vi "status_machine_value.vi"(8 "Main_Status_in":T2, 9 "Main상태쓰기":bool, 10 "Vesa_Status_in":T1, 11 "vesa상태쓰기":bool) -> (0 "Main Exit?":bool, 1 "Main_Status":T2, 2 "DisConnect?":bool, 3 "Vesa_Status":T1)   [LabVIEW 2014]
uses:
  VESA_Status.ctl
  Main_status.ctl
  bus_button.xctl
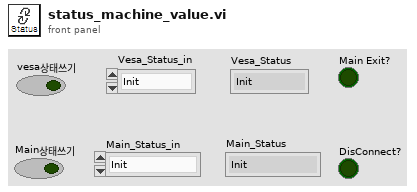
[diagram p1: front panel]
types:
  T1 = typedef "bus_button.xctl/VESA_Status.ctl" = enum16{"Init", "Wait", "Connect", "DisConnect", "Idel", "Exit"}
  T2 = typedef "Main_status.ctl" = enum16{"Init", "Wait", "connect", "Idle", "disc", "Exit"}
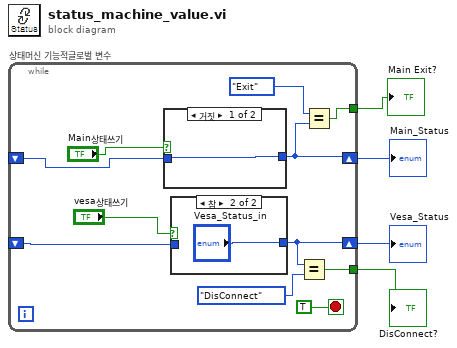
[diagram p0: block diagram]
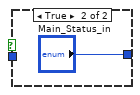
[diagram p2: hidden frame]
diagram:
  n1 = while "상태머신 기능적글로벌 변수" {
    shift-right: [w7] -> w4
    shift-left: _ -> [w12]
    shift-right: [w10] -> w3
    shift-left: _ -> [w14]
    tunnel: [w8] -> w2
    tunnel: [w5] -> w1
    stop <- TRUE stop-if-true
    n2 = case shown="거짓" "Main상태쓰기" {
      tunnel: [w16 "Main_Status_in"] -> w7
      tunnel: w12 -> [w16 _]
      frame False {
      }
      frame True {
      }
    }
    n3 = case shown="참" "vesa상태쓰기" {
      tunnel: [w18 "Vesa_Status_in"] -> w10
      tunnel: w14 -> [w18 _]
      frame False {
      }
      frame True {
      }
    }
    n4 = Equal?(x=w10, y=VESA_Status."DisConnect") -> (x = y?=w8:bool)
    n5 = Equal?(x=Main_status."Exit" ("Main_Status"), y=w7) -> (x = y?=w5:bool)
  }
  "Main_Status" <- w4
  "Vesa_Status" <- w3
  "DisConnect?" <- w2
  "Main Exit?" <- w1
